vi "Initialize Attributes.vi"(8 "error in (no error)":errorcluster, 10 "Attribute Data":variant, 11 "CS++Fgen in":refnum<class "CS++Fgen.lvclass">) -> (0 "error out":errorcluster, 2 "Found?":bool, 3 "CS++Fgen out":refnum<class "CS++Fgen.lvclass">)   [LabVIEW 2013, in "CS++Fgen.lvlib" / "CS++Fgen.lvclass"]
doc: "Initialize object attribute.\n\nUnique resources should be allocated elsewhere!"
uses:
  CS++Fgen.lvclass
  Core/Actors/CS++DeviceActor/CS++DeviceActor.lvclass
  Core/Actors/CS++BaseActor/CS++BaseActor.lvclass/CS++BaseActor.ctl
  Core/Classes/CS++BaseClasses/Factory/CS++Factory.lvclass
  CS++Fgen.lvclass/CS++Fgen.ctl
  Core/Actors/CS++BaseActor/CS++BaseActor.lvclass
  Core/Libraries/Utilities/CS++Utilities.lvlib
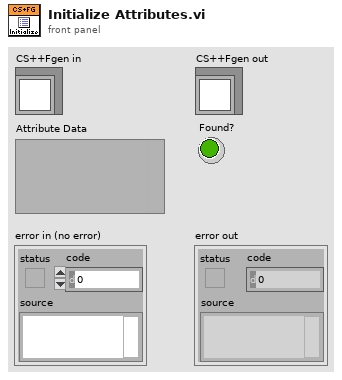
[diagram p1: front panel]
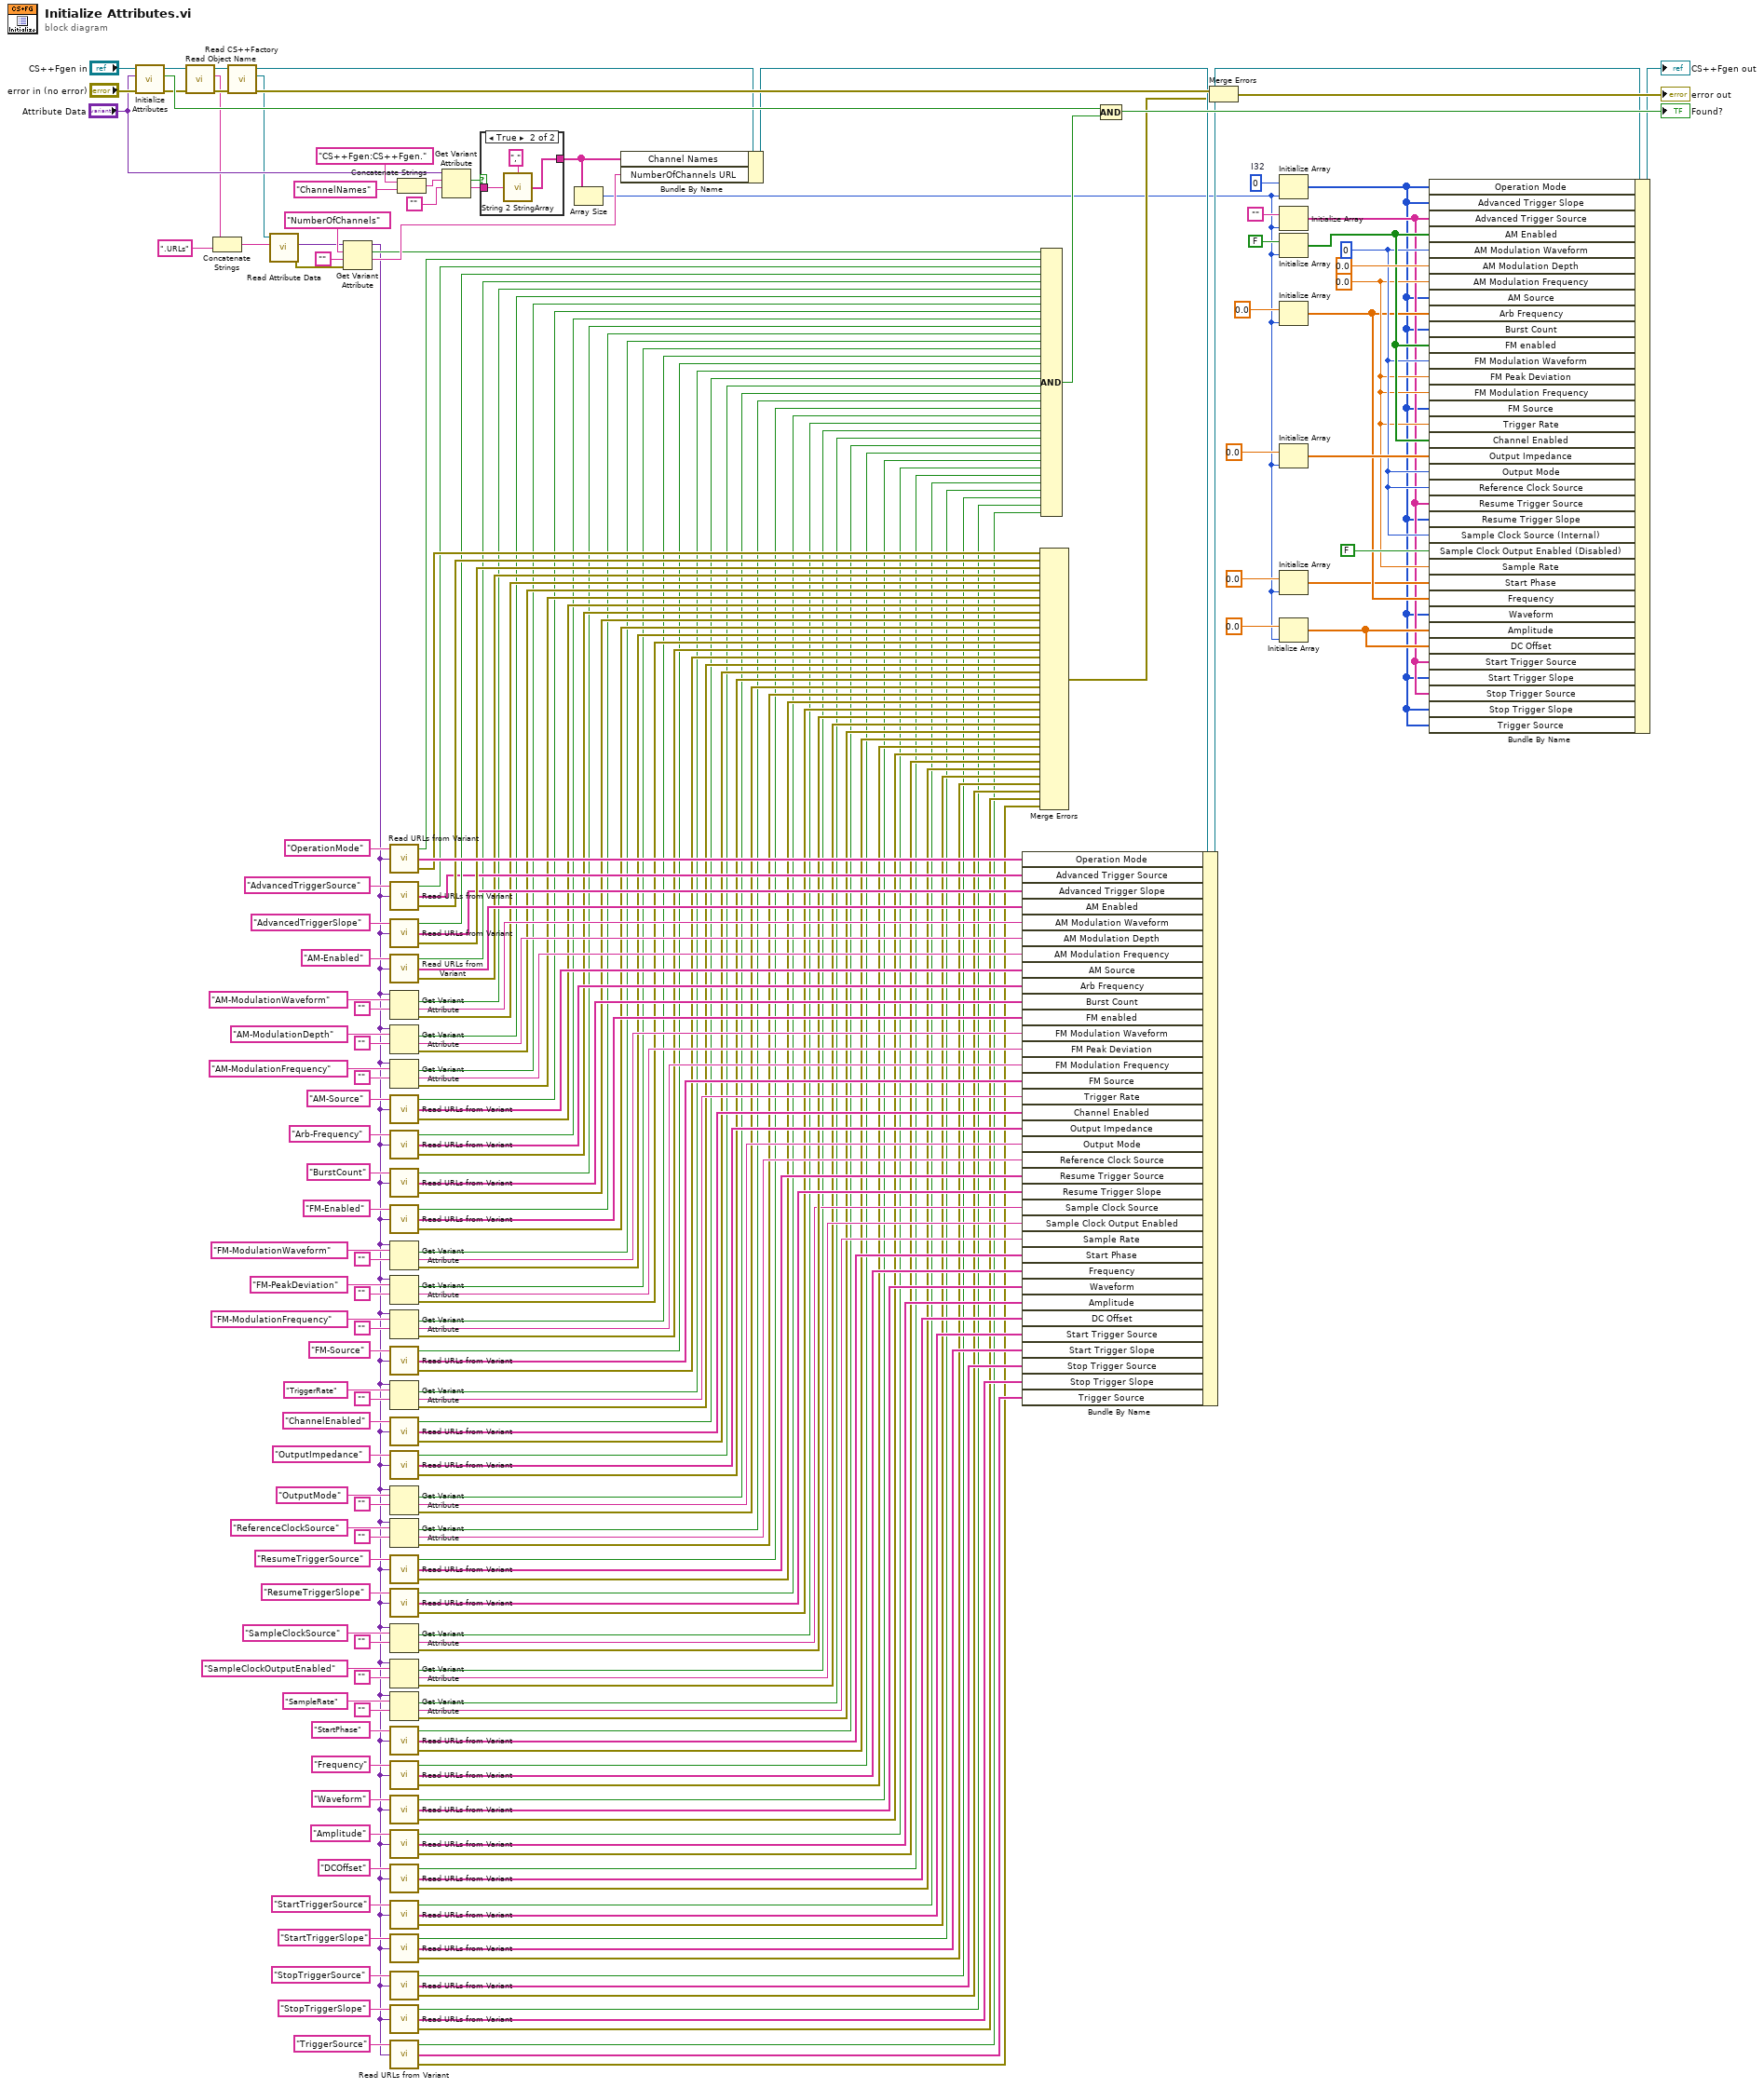
[diagram p0: block diagram]
diagram:
  w50 = dbl[unit] 0.0 ("modulation depth (0.00 %)")
  w67 = 0 ("I32")
  w170 = 0  # I32
  n1 = call-parent "Initialize Attributes.vi"("error in (no error)"="error in (no error)", "Attribute Data"="Attribute Data", "CS++DeviceActor in"="CS++Fgen in") -> ("error out"=w200:errorcluster, "Found?"=w204:bool, "CS++DeviceActor out"=w202:refnum<class "CS++Fgen.lvclass">)  [unwired: 6 in]
  n2 = call "Read Object Name.vi"("error in (no error)"=w200, "CS++BaseActor in"=w202) -> ("error out"=w201:errorcluster, "Object Name"=w180:string, "CS++BaseActor out"=w203:refnum<class "CS++Fgen.lvclass">)  [unwired: 7 in]
  n3 = Concatenate Strings(w180, ".URLs" ("string")) -> (w185:string)
  n4 = call "Read CS++Factory.vi"("error in (no error)"=w201, "CS++BaseActor in"=w203) -> ("error out"=w199:errorcluster, "CS++Factory"=w183:refnum<class "CS++Factory.lvclass">, "CS++BaseActor out"=w191:refnum<class "CS++Fgen.lvclass">)  [unwired: 7 in]
  n5 = call-dynamic "Read Attribute Data.vi"("Object Name"=w185, "CS++Factory in"=w183) -> ("error out"=w186:errorcluster, "Attribute Data"=w187:variant)  [unwired: 7 in, 1 out]
  n6 = Get Variant Attribute(Variant=w187, name="NumberOfChannels" ("string"), default value (empty Variant)="", error in=w186) -> (duplicate Variant=w4:variant, found=w171:bool, value=w182:string)  [unwired: 1 out]
  n7 = call "Read URLs from Variant.vi"("URL Section Data"=w4, "URL Prefix"="OperationMode" ("string")) -> ("Error Out"=w175:errorcluster, "URLs"=w177:string[], "Found?"=w173:bool)  [unwired: 1 in]
  n8 = call "Read URLs from Variant.vi"("URL Section Data"=w4, "URL Prefix"="AdvancedTriggerSource" ("string")) -> ("Error Out"=w164:errorcluster, "URLs"=w161:string[], "Found?"=w165:bool)  [unwired: 1 in]
  n9 = call "Read URLs from Variant.vi"("URL Section Data"=w4, "URL Prefix"="AdvancedTriggerSlope" ("string")) -> ("Error Out"=w162:errorcluster, "URLs"=w160:string[], "Found?"=w163:bool)  [unwired: 1 in]
  n10 = call "Read URLs from Variant.vi"("URL Section Data"=w4, "URL Prefix"="AM-Enabled" ("string")) -> ("Error Out"=w156:errorcluster, "URLs"=w157:string[], "Found?"=w158:bool)  [unwired: 1 in]
  n11 = Get Variant Attribute(Variant=w4, name="AM-ModulationWaveform", default value (empty Variant)="") -> (found=w150:bool, value=w151:string, error out=w149:errorcluster)  [unwired: 1 in, 1 out]
  n12 = Get Variant Attribute(Variant=w4, name="AM-ModulationDepth", default value (empty Variant)="") -> (found=w144:bool, value=w143:string, error out=w142:errorcluster)  [unwired: 1 in, 1 out]
  n13 = Get Variant Attribute(Variant=w4, name="AM-ModulationFrequency", default value (empty Variant)="") -> (found=w141:bool, value=w140:string, error out=w139:errorcluster)  [unwired: 1 in, 1 out]
  n14 = call "Read URLs from Variant.vi"("URL Section Data"=w4, "URL Prefix"="AM-Source" ("string")) -> ("Error Out"=w134:errorcluster, "URLs"=w135:string[], "Found?"=w136:bool)  [unwired: 1 in]
  n15 = call "Read URLs from Variant.vi"("URL Section Data"=w4, "URL Prefix"="Arb-Frequency" ("string")) -> ("Error Out"=w130:errorcluster, "URLs"=w131:string[], "Found?"=w132:bool)  [unwired: 1 in]
  n16 = call "Read URLs from Variant.vi"("URL Section Data"=w4, "URL Prefix"="BurstCount" ("string")) -> ("Error Out"=w125:errorcluster, "URLs"=w126:string[], "Found?"=w127:bool)  [unwired: 1 in]
  n17 = call "Read URLs from Variant.vi"("URL Section Data"=w4, "URL Prefix"="FM-Enabled" ("string")) -> ("Error Out"=w121:errorcluster, "URLs"=w122:string[], "Found?"=w123:bool)  [unwired: 1 in]
  n18 = Get Variant Attribute(Variant=w4, name="FM-ModulationWaveform", default value (empty Variant)="") -> (found=w114:bool, value=w113:string, error out=w112:errorcluster)  [unwired: 1 in, 1 out]
  n19 = Get Variant Attribute(Variant=w4, name="FM-PeakDeviation", default value (empty Variant)="") -> (found=w111:bool, value=w110:string, error out=w109:errorcluster)  [unwired: 1 in, 1 out]
  n20 = Get Variant Attribute(Variant=w4, name="FM-ModulationFrequency", default value (empty Variant)="") -> (found=w108:bool, value=w107:string, error out=w106:errorcluster)  [unwired: 1 in, 1 out]
  n21 = call "Read URLs from Variant.vi"("URL Section Data"=w4, "URL Prefix"="FM-Source" ("string")) -> ("Error Out"=w102:errorcluster, "URLs"=w103:string[], "Found?"=w104:bool)  [unwired: 1 in]
  n22 = Get Variant Attribute(Variant=w4, name="TriggerRate", default value (empty Variant)="") -> (found=w99:bool, value=w98:string, error out=w97:errorcluster)  [unwired: 1 in, 1 out]
  n23 = call "Read URLs from Variant.vi"("URL Section Data"=w4, "URL Prefix"="ChannelEnabled" ("string")) -> ("Error Out"=w93:errorcluster, "URLs"=w94:string[], "Found?"=w95:bool)  [unwired: 1 in]
  n24 = call "Read URLs from Variant.vi"("URL Section Data"=w4, "URL Prefix"="OutputImpedance" ("string")) -> ("Error Out"=w88:errorcluster, "URLs"=w89:string[], "Found?"=w90:bool)  [unwired: 1 in]
  n25 = Get Variant Attribute(Variant=w4, name="OutputMode", default value (empty Variant)="") -> (found=w83:bool, value=w82:string, error out=w81:errorcluster)  [unwired: 1 in, 1 out]
  n26 = Get Variant Attribute(Variant=w4, name="ReferenceClockSource", default value (empty Variant)="") -> (found=w78:bool, value=w77:string, error out=w76:errorcluster)  [unwired: 1 in, 1 out]
  n27 = call "Read URLs from Variant.vi"("URL Section Data"=w4, "URL Prefix"="ResumeTriggerSource" ("string")) -> ("Error Out"=w71:errorcluster, "URLs"=w72:string[], "Found?"=w73:bool)  [unwired: 1 in]
  n28 = call "Read URLs from Variant.vi"("URL Section Data"=w4, "URL Prefix"="ResumeTriggerSlope" ("string")) -> ("Error Out"=w68:errorcluster, "URLs"=w69:string[], "Found?"=w70:bool)  [unwired: 1 in]
  n29 = Get Variant Attribute(Variant=w4, name="SampleClockSource", default value (empty Variant)="") -> (found=w64:bool, value=w62:string, error out=w63:errorcluster)  [unwired: 1 in, 1 out]
  n30 = Get Variant Attribute(Variant=w4, name="SampleClockOutputEnabled", default value (empty Variant)="") -> (found=w58:bool, value=w57:string, error out=w56:errorcluster)  [unwired: 1 in, 1 out]
  n31 = Get Variant Attribute(Variant=w4, name="SampleRate", default value (empty Variant)="") -> (found=w53:bool, value=w52:string, error out=w51:errorcluster)  [unwired: 1 in, 1 out]
  n32 = call "Read URLs from Variant.vi"("URL Section Data"=w4, "URL Prefix"="StartPhase" ("string")) -> ("Error Out"=w36:errorcluster, "URLs"=w37:string[], "Found?"=w38:bool)  [unwired: 1 in]
  n33 = call "Read URLs from Variant.vi"("URL Section Data"=w4, "URL Prefix"="Frequency" ("string")) -> ("Error Out"=w33:errorcluster, "URLs"=w34:string[], "Found?"=w35:bool)  [unwired: 1 in]
  n34 = call "Read URLs from Variant.vi"("URL Section Data"=w4, "URL Prefix"="Waveform" ("string")) -> ("Error Out"=w30:errorcluster, "URLs"=w31:string[], "Found?"=w32:bool)  [unwired: 1 in]
  n35 = call "Read URLs from Variant.vi"("URL Section Data"=w4, "URL Prefix"="Amplitude" ("string")) -> ("Error Out"=w27:errorcluster, "URLs"=w28:string[], "Found?"=w29:bool)  [unwired: 1 in]
  n36 = call "Read URLs from Variant.vi"("URL Section Data"=w4, "URL Prefix"="DCOffset" ("string")) -> ("Error Out"=w24:errorcluster, "URLs"=w25:string[], "Found?"=w26:bool)  [unwired: 1 in]
  n37 = call "Read URLs from Variant.vi"("URL Section Data"=w4, "URL Prefix"="StartTriggerSource" ("string")) -> ("Error Out"=w19:errorcluster, "URLs"=w20:string[], "Found?"=w21:bool)  [unwired: 1 in]
  n38 = call "Read URLs from Variant.vi"("URL Section Data"=w4, "URL Prefix"="StartTriggerSlope" ("string")) -> ("Error Out"=w16:errorcluster, "URLs"=w17:string[], "Found?"=w18:bool)  [unwired: 1 in]
  n39 = call "Read URLs from Variant.vi"("URL Section Data"=w4, "URL Prefix"="StopTriggerSource" ("string")) -> ("Error Out"=w11:errorcluster, "URLs"=w12:string[], "Found?"=w13:bool)  [unwired: 1 in]
  n40 = call "Read URLs from Variant.vi"("URL Section Data"=w4, "URL Prefix"="StopTriggerSlope" ("string")) -> ("Error Out"=w8:errorcluster, "URLs"=w9:string[], "Found?"=w10:bool)  [unwired: 1 in]
  n41 = call "Read URLs from Variant.vi"("URL Section Data"=w4, "URL Prefix"="TriggerSource" ("string")) -> ("Error Out"=w1:errorcluster, "URLs"=w2:string[], "Found?"=w3:bool)  [unwired: 1 in]
  n42 = Concatenate Strings("CS++Fgen:CS++Fgen.", "ChannelNames" ("string")) -> (w194:string)
  n43 = Get Variant Attribute(Variant="Attribute Data", name=w194, default value (empty Variant)="") -> (found=w197:bool, value=w196:string)  [unwired: 1 in, 2 out]
  n44 = case shown="True" w197 {
    tunnel: w196 -> [_ w209]
    tunnel: [_ w208] -> w190
    frame False {
    }
    frame True {
      n45 = call "String 2 StringArray.vi"("String"=w209, "Delimiter (\",\")"="," ("Delimiter (\",\")")) -> ("Substrings"=w208:string[])
    }
  }
  n46 = Array Size(array=w190) -> (size(s)=w45:i32)
  n47 = Bundle By Name(cluster=w191, "Channel Names"=w190, "NumberOfChannels URL"=w182) -> (w178:refnum<class "CS++Fgen.lvclass">)
  n48 = Bundle By Name(cluster=w178, "Operation Mode"=w177, "Advanced Trigger Source"=w161, "Advanced Trigger Slope"=w160, "AM Enabled"=w157, "AM Modulation Waveform"=w151, "AM Modulation Depth"=w143, "AM Modulation Frequency"=w140, "AM Source"=w135, "Arb Frequency"=w131, "Burst Count"=w126, "FM enabled"=w122, "FM Modulation Waveform"=w113, "FM Peak Deviation"=w110, "FM Modulation Frequency"=w107, "FM Source"=w103, "Trigger Rate"=w98, "Channel Enabled"=w94, "Output Impedance"=w89, "Output Mode"=w82, "Reference Clock Source"=w77, "Resume Trigger Source"=w72, "Resume Trigger Slope"=w69, "Sample Clock Source"=w62, "Sample Clock Output Enabled"=w57, "Sample Rate"=w52, "Start Phase"=w37, "Frequency"=w34, "Waveform"=w31, "Amplitude"=w28, "DC Offset"=w25, "Start Trigger Source"=w20, "Start Trigger Slope"=w17, "Stop Trigger Source"=w12, "Stop Trigger Slope"=w9, "Trigger Source"=w2) -> (w169:refnum<class "CS++Fgen.lvclass">)
  n49 = Merge Errors(w175, w164, w162, w156, w149, w142, w139, w134, w130, w125, w121, w112, w109, w106, w102, w97, w93, w88, w81, w76, w71, w68, w63, w56, w51, w36, w33, w30, w27, w24, w19, w16, w11, w8, w1) -> (w174:errorcluster)
  n50 = Compound Arithmetic op=AND(w171, w173, w165, w163, w158, w150, w144, w141, w136, w132, w127, w123, w114, w111, w108, w104, w99, w95, w90, w83, w78, w73, w70, w64, w58, w53, w38, w35, w32, w29, w26, w21, w18, w13, w10, w3) -> (w172:bool)
  n51 = Compound Arithmetic op=AND(w204, w172) -> (→"Found?":bool)
  n52 = Merge Errors(w199, w174) -> (→"error out":errorcluster)
  n53 = Initialize Array(w170, w45) -> (w6:i32[])
  n54 = Initialize Array("" ("output state (Constant Voltage)"), w45) -> (w7:string[])
  n55 = Initialize Array(FALSE, w45) -> (w92:bool[])
  n56 = Initialize Array(dbl[unit] 0.0 ("modulation depth (0.00 %)"), w45) -> (w49:dbl[unit][])
  n57 = Initialize Array(dbl[unit] 0.0 ("modulation depth (0.00 %)"), w45) -> (w86:dbl[unit][])
  n58 = Initialize Array(dbl[unit] 0.0 ("modulation depth (0.00 %)"), w45) -> (w47:dbl[unit][])
  n59 = Initialize Array(dbl[unit] 0.0 ("modulation depth (0.00 %)"), w45) -> (w44:dbl[unit][])
  n60 = Bundle By Name(cluster=w169, "Operation Mode"=w6, "Advanced Trigger Slope"=w6, "Advanced Trigger Source"=w7, "AM Enabled"=w92, "AM Modulation Waveform"=w67, "AM Modulation Depth"=0.0 ("modulation depth (0.00 %)"), "AM Modulation Frequency"=w50, "AM Source"=w6, "Arb Frequency"=w49, "Burst Count"=w6, "FM enabled"=w92, "FM Modulation Waveform"=w67, "FM Peak Deviation"=w50, "FM Modulation Frequency"=w50, "FM Source"=w6, "Trigger Rate"=w50, "Channel Enabled"=w92, "Output Impedance"=w86, "Output Mode"=w67, "Reference Clock Source"=w67, "Resume Trigger Source"=w7, "Resume Trigger Slope"=w6, "Sample Clock Source (Internal)"=w67, "Sample Clock Output Enabled (Disabled)"=FALSE, "Sample Rate"=w50, "Start Phase"=w47, "Frequency"=w49, "Waveform"=w6, "Amplitude"=w44, "DC Offset"=w44, "Start Trigger Source"=w7, "Start Trigger Slope"=w6, "Stop Trigger Source"=w7, "Stop Trigger Slope"=w6, "Trigger Source"=w6) -> (→"CS++Fgen out":refnum<class "CS++Fgen.lvclass">)
